vi "Main.vi"() -> ()   [LabVIEW 2018]
doc: "This Continuous Measurement sample project is based on the Queued Message Handler template.\n\nThe Event Handling Loop generates messages based on user interface actions.\n\nThe Message Handling Loop processes messages generated by the Event Handling Loop, or by other messages. There are also Acquisition and Logging message handling loop subVIs, and a chart updating loop."
uses:
  Settings/Settings.ctl
  Acquisition/Hardware Configuration.ctl
  Logging/Logging Configuration.ctl
  controls/UI Data.ctl
  controls/UI State.ctl
  support/Message Queue/Enqueue Message (Single).vi
  support/Message Queue/Enqueue Message (Array).vi
  <vilib>/Utility/error.llb/Error Cluster From Error Code.vi
  <vilib>/ErrorRing/Error Ring.xnode
  Acquisition/Acquisition.lvlib
  Logging/Logging.lvlib
  Settings/Settings.lvlib
  support/User Event - Stop/User Event - Stop.lvlib
  support/Message Queue/Message Queue.lvlib
  Settings/Settings Dialog.vi
panel:
  in  "Data 2":u32(graph)
  out "Config":T1={"Hardware Configuration"={"DAQmx Channel 1"="SimDev1/ai0", "DAQmx Channel 2"="SimDev1/ai1", "DAQmx Channel 3"="SimDev1/ai2", "DAQmx AI Task"="", "Channel 1 Name"="Battery Voltage", "Channel 2 Name"="Battery Current", "Channel 3 Name"="Brake torque", "Sample time"=50, "Samples per second"=1000.0, "Sample mode"=0, "Samples per channel"=0, "Offset Channel 1"=0.0, "Offset Channel 2"=0.0, "Offset Channel 3"=0.0, "Scale Channel 1"=0.0, "Scale Channel 2"=0.0, "Scale Channel 3"=0.0, "DAQmx Counter Channel"="", "Counter Name"="", "DAQmx Counter Task"=""}, "Logging Configuration"={"Log File Base Path"=path "", "TDMS File Reference"=refnum}} {"Hardware Configuration"."Sample mode" items=["Continuous Samples"=10123]}
  out "Data":u32(graph)
  in  "Start":bool
  in  "Stop":bool
  in  "Settings":bool
  out "Status":string
  in  "data to matlab":bool
  in  "Exit":bool
  # "Scooter measurement data"
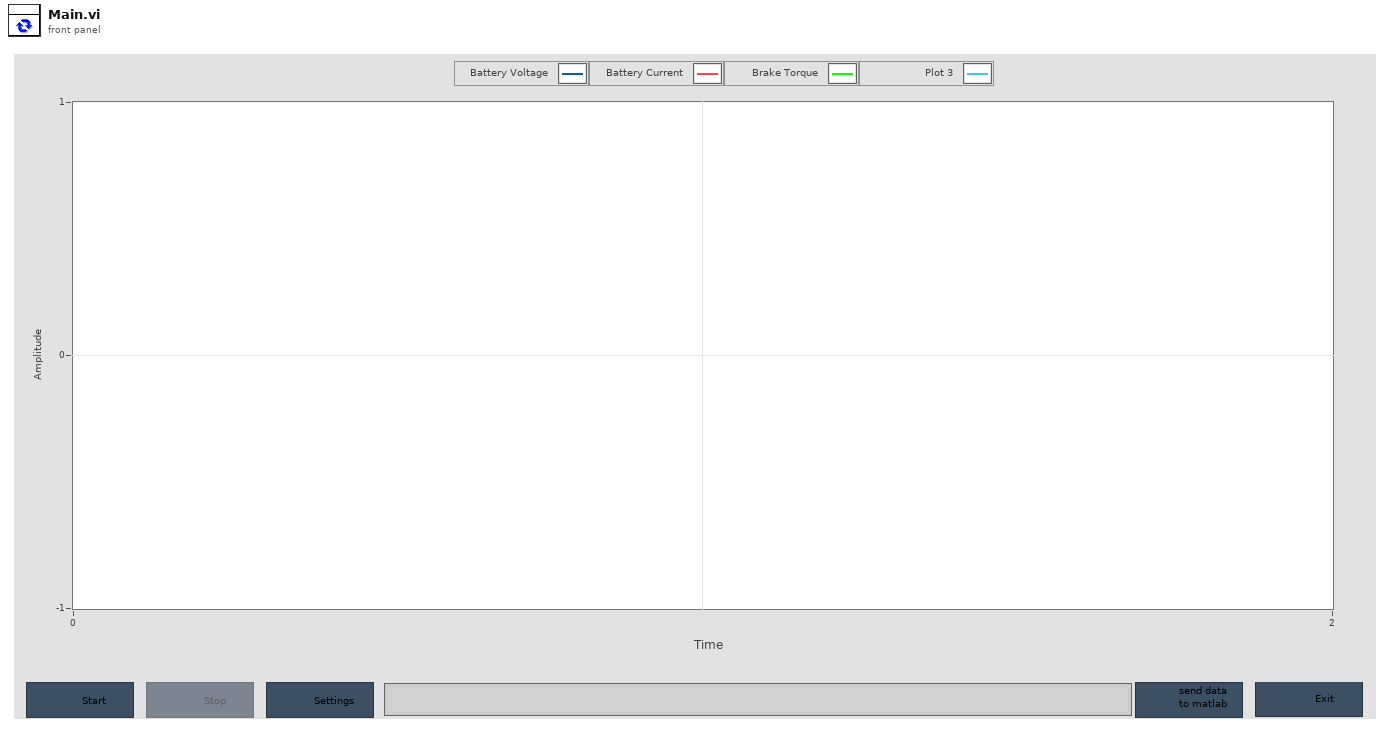
[diagram p1: front panel]
types:
  T1 = typedef "Settings.lvlib/Settings.ctl" = cluster{"Hardware Configuration":T2, "Logging Configuration":T3}
  T2 = typedef "Acquisition.lvlib/Hardware Configuration.ctl" = cluster{"DAQmx Channel 1":tag, "DAQmx Channel 2":tag, "DAQmx Channel 3":tag, "DAQmx AI Task":refnum<k21>, "Channel 1 Name":string, "Channel 2 Name":string, "Channel 3 Name":string, "Sample time":u32, "Samples per second":dbl, "Sample mode":u16, "Samples per channel":i32, "Offset Channel 1":dbl, "Offset Channel 2":dbl, "Offset Channel 3":dbl, "Scale Channel 1":dbl, "Scale Channel 2":dbl, "Scale Channel 3":dbl, "DAQmx Counter Channel":tag, "Counter Name":string, "DAQmx Counter Task":refnum<k21>}
  T3 = typedef "Logging.lvlib/Logging Configuration.ctl" = cluster{"Log File Base Path":path, "TDMS File Reference":refnum<k34>}
  T4 = typedef "UI State.ctl" = enum16{"Idle", "Acquiring and Logging", "Waiting for Exit", "Waiting for Exit (Acq Stopped)", "Waiting for Exit (Log Stopped)", "Waiting for Stop", "Waiting for Stop (Acq Stopped)", "Waiting for Stop (Log Stopped)"}
  T5 = typedef "UI Data.ctl" = cluster{"Start Ref":refnum<vi>, "Stop Ref":refnum<vi>, "Settings Ref":refnum<vi>, "Exit Ref":refnum<vi>, "Status Ref":refnum<vi>, "Data Ref":refnum<vi>, "data to matlab Ref":refnum<vi>}
  T6 = typedef "Message Queue.lvlib/All Message Queues.ctl" = cluster{"UI":refnum<queue>, "Acquisition":refnum<queue>, "Logging":refnum<queue>}
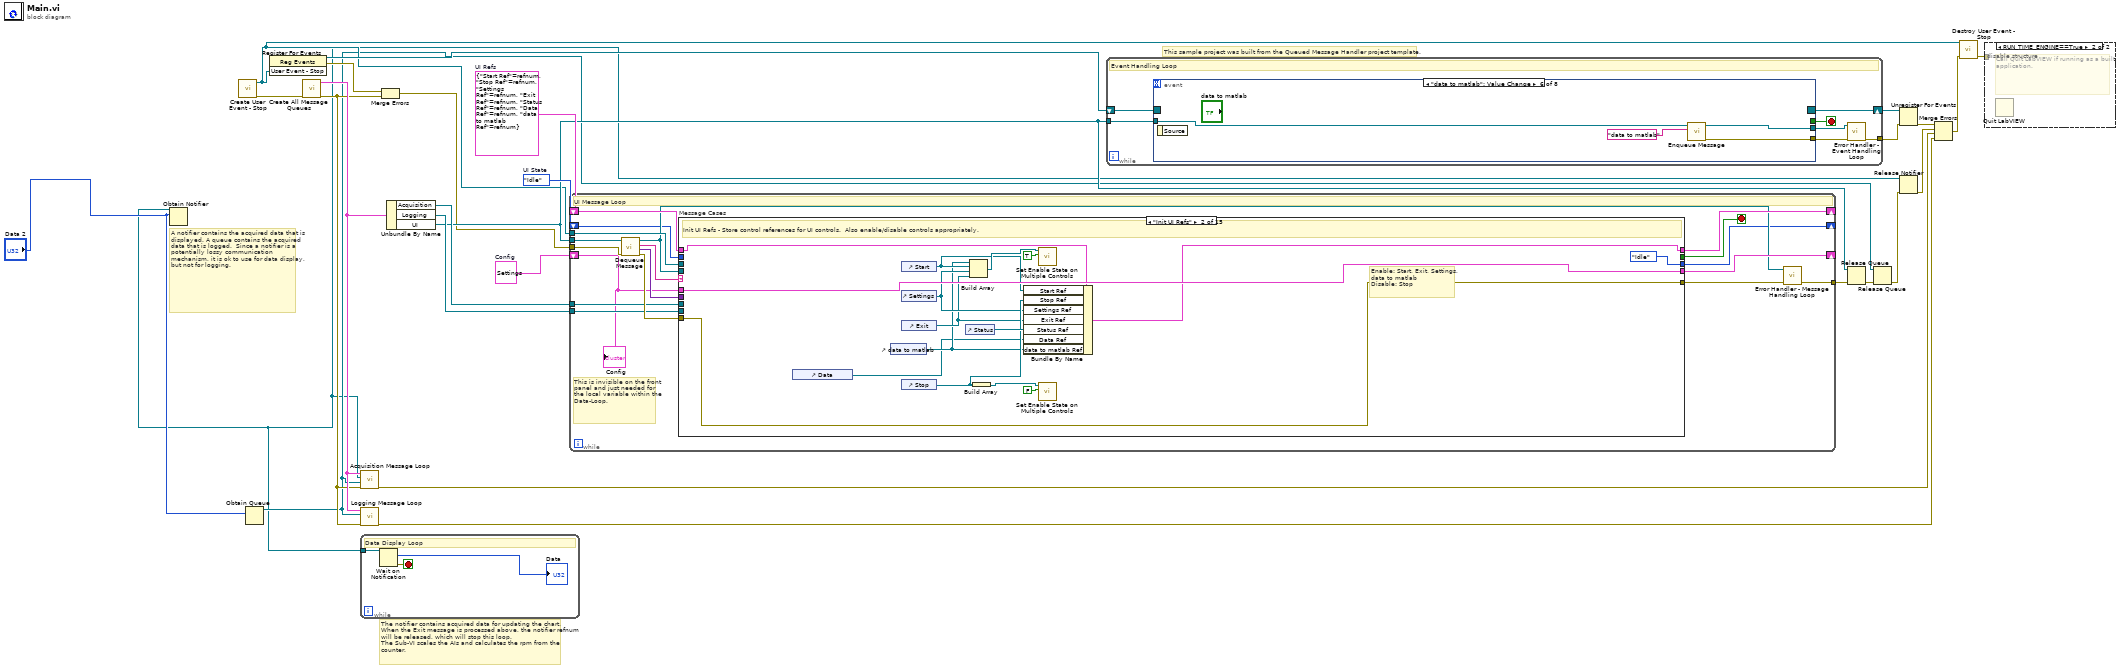
[diagram p0: block diagram]
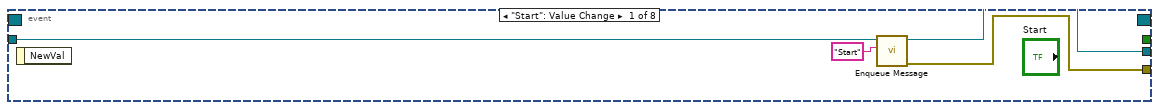
[diagram p3: hidden frame]
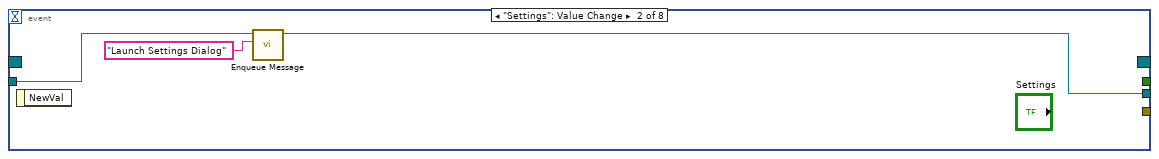
[diagram p4: hidden frame]
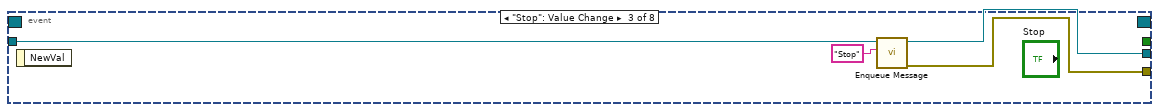
[diagram p5: hidden frame]
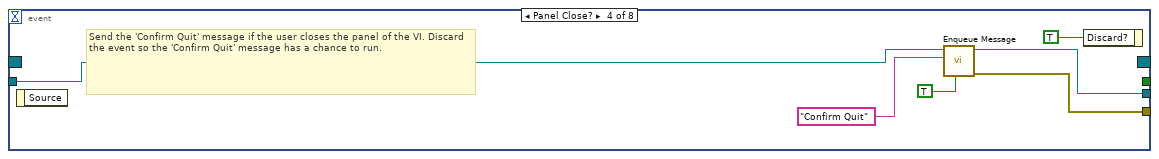
[diagram p6: hidden frame]
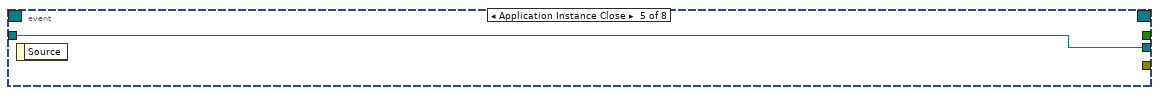
[diagram p7: hidden frame]
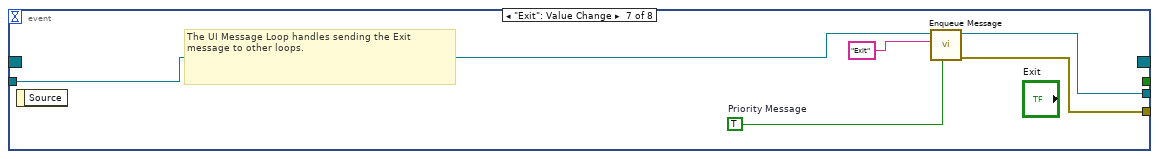
[diagram p8: hidden frame]
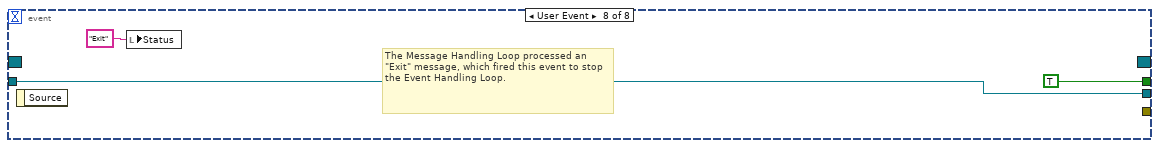
[diagram p9: hidden frame]
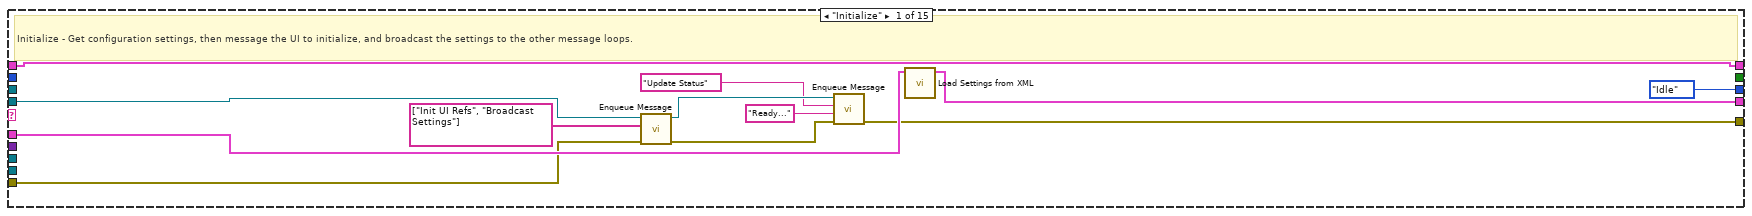
[diagram p10: hidden frame]
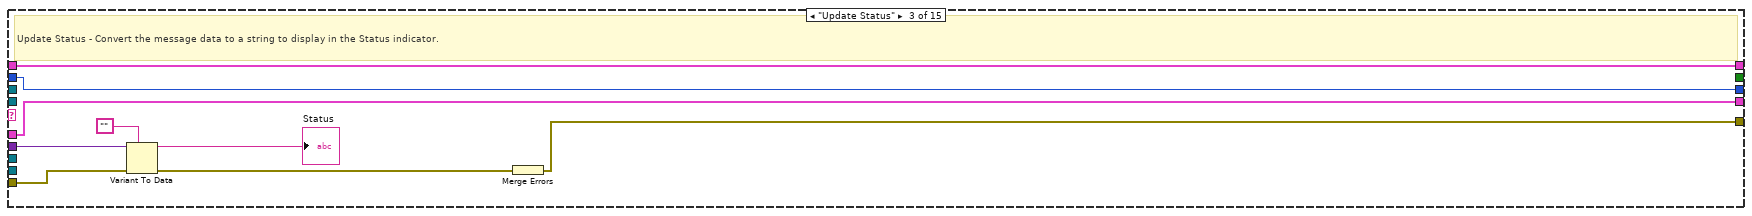
[diagram p11: hidden frame]
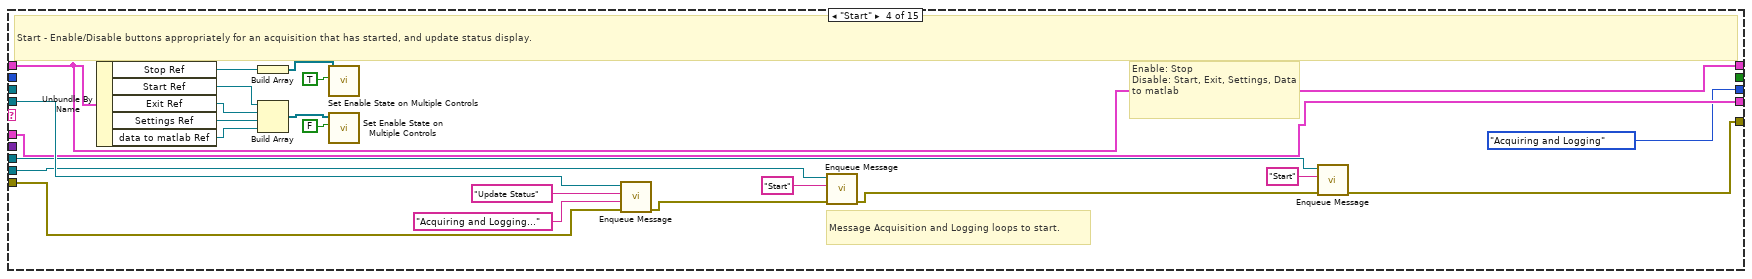
[diagram p12: hidden frame]
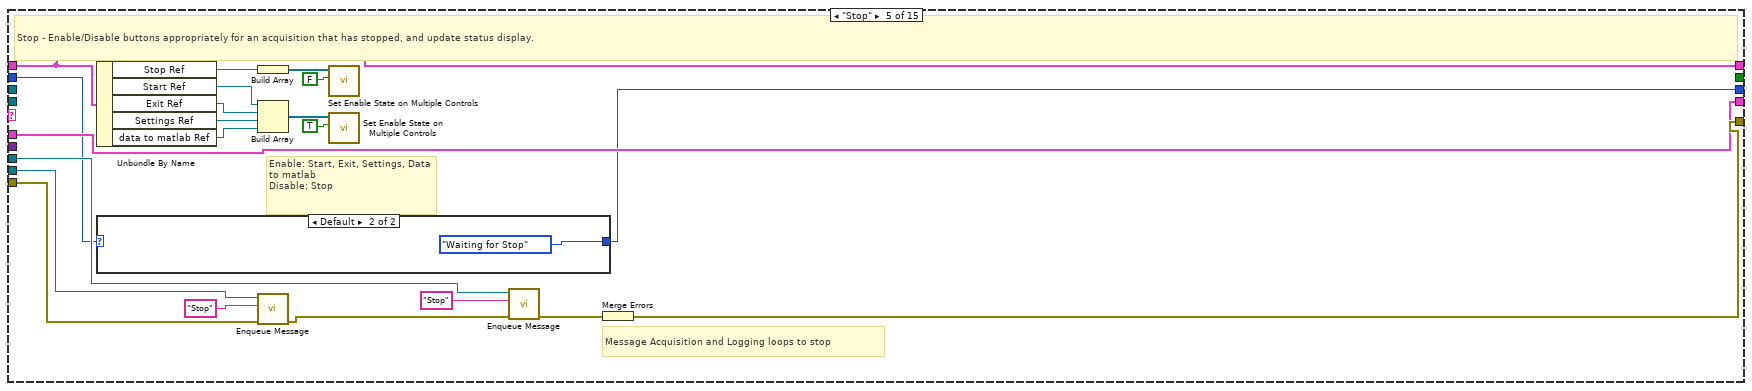
[diagram p13: hidden frame]
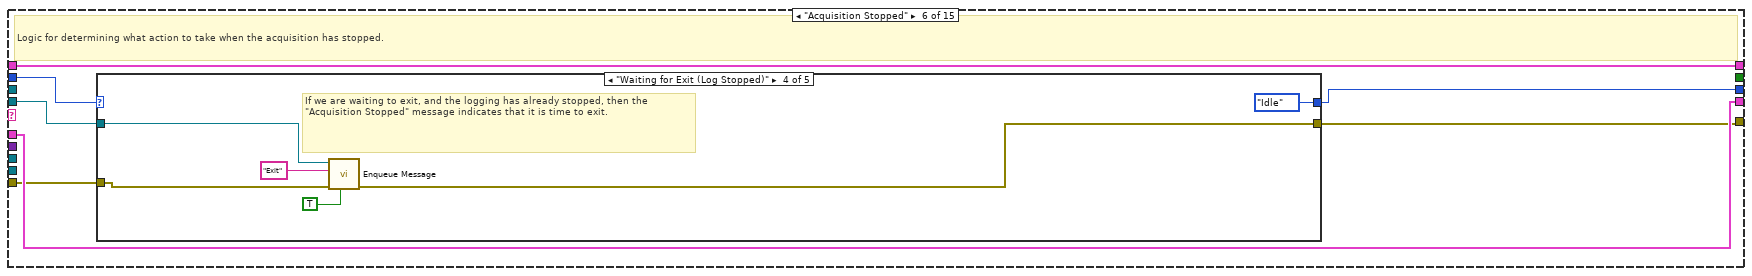
[diagram p15: hidden frame]
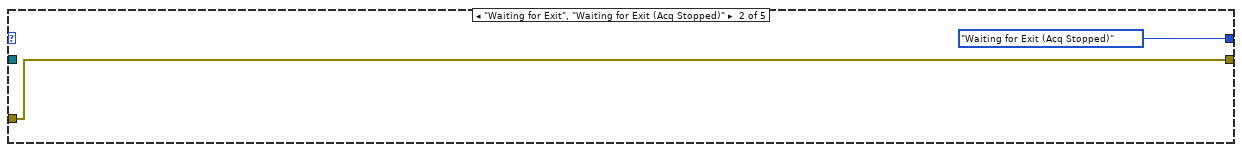
[diagram p17: hidden frame]
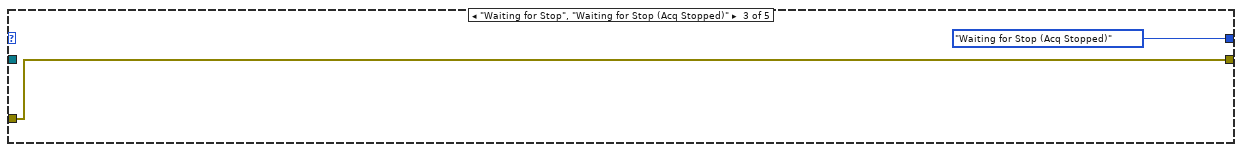
[diagram p18: hidden frame]
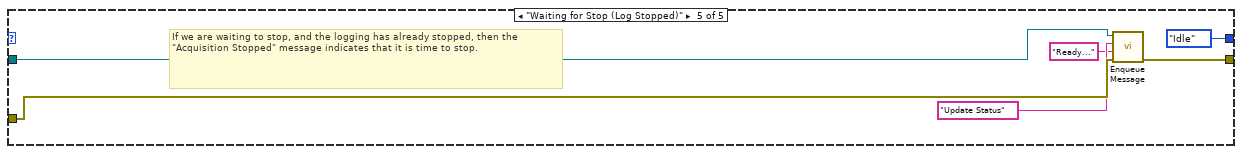
[diagram p19: hidden frame]
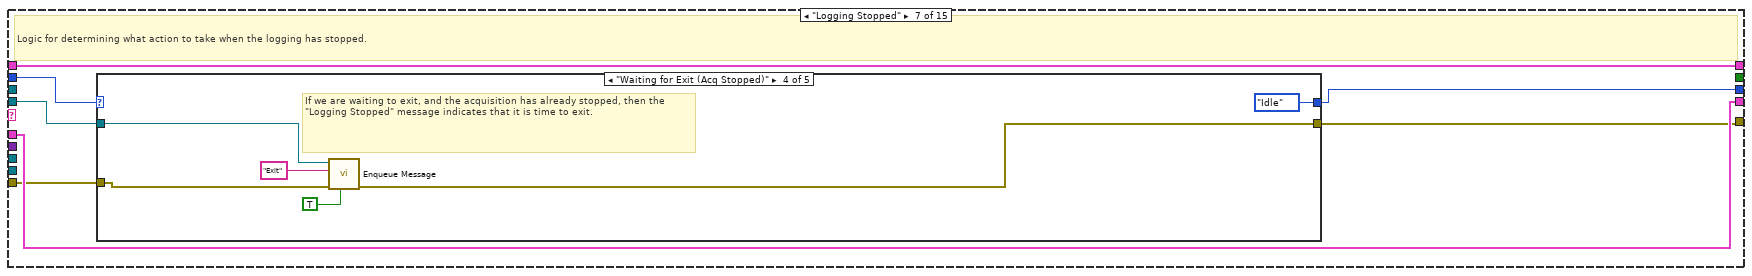
[diagram p20: hidden frame]
diagram:
  w15 = UI_State."Idle"  # UI State
  w18 = T5 {"Start Ref"=refnum, "Stop Ref"=refnum, "Settings Ref"=refnum, "Exit Ref"=refnum, "Status Ref"=refnum, "Data Ref"=refnum, "data to matlab Ref"=refnum}  # UI Refs
  w4 = T1 {"Hardware Configuration"={"DAQmx Channel 1"="", "DAQmx Channel 2"="", "DAQmx Channel 3"="", "DAQmx AI Task"="", "Channel 1 Name"="Battery Voltage", "Channel 2 Name"="Battery Current", "Channel 3 Name"="Brake torque", "Sample time"=50, "Samples per second"=1000.0, "Sample mode"=0, "Samples per channel"=0, "Offset Channel 1"=0.0, "Offset Channel 2"=0.0, "Offset Channel 3"=0.0, "Scale Channel 1"=0.0, "Scale Channel 2"=0.0, "Scale Channel 3"=0.0, "DAQmx Counter Channel"="", "Counter Name"="", "DAQmx Counter Task"=""}, "Logging Configuration"={"Log File Base Path"=path "", "TDMS File Reference"=refnum}}  # Config
  # "This sample project was built from the Queued Message Handler project template."
  # "A notifier contains the acquired data that is displayed. A queue contains the acquired data that is logged.  Since a notifier is a potentially lossy communication mechanism, it is ok to use for data display, but not for logging."
  # "The notifier contains acquired data for updating the chart. When the Exit message is processed above, the notifier refnum will be released, which will stop this loop.\nThe Sub-VI scales the AIs and calculates the rpm from the counter."
  n1 = Obtain Notifier(notification data type="Data 2") -> (notifier out=w1:refnum<notifier>)  [unwired: 3 in, 2 out]
  n2 = call "Create User Event - Stop.vi"() -> ("error out"=w24:errorcluster, "User Event - Stop"=w7:refnum<user-event>)  [unwired: 10 in]
  n3 = Obtain Queue(element data type="Data 2") -> (queue out=w2:refnum<queue>)  [unwired: 4 in, 2 out]
  n4 = register-events(w7) -> (reference out=w8:refnum<event-registration>, error out=w5:errorcluster)  [unwired: 2 in]
  n5 = call "Create All Message Queues.vi"("error in (no error)"=w24) -> ("error out"=w21:errorcluster, "Message Queues out"=w23:T6)  [unwired: 9 in]
  n6 = call "Acquisition Message Loop.vi"("error in (no error)"=w21, "Data Queue"=w2, "Data Notifier"=w1, "Message Queues"=w23) -> ("error out"=w25:errorcluster)  [unwired: 7 in]
  n7 = call "Logging Message Loop.vi"("error in (no error)"=w21, "Data Queue"=w2, "Message Queues"=w23) -> ("error out"=w22:errorcluster)  [unwired: 8 in]
  n8 = while "Data Display Loop" {
    tunnel: w1 -> [w30]
    stop <- w29 stop-if-true
    # "Data Display Loop"
    n9 = Wait on Notification(notifier=w30) -> (notification=→"Data":u32, error out=w29:errorcluster)  [unwired: 3 in, 2 out]
  }
  n10 = Merge Errors(w5, w21) -> (w6:errorcluster)
  n11 = Unbundle By Name(w23) -> ("Acquisition"=w17:refnum<queue>, "Logging"=w16:refnum<queue>, "UI"=w13:refnum<queue>)
  n12 = while {
    tunnel: w13 -> [w42]
    tunnel: w7 -> [w47]
    shift-right: [w41] -> _
    shift-left: w4 -> [w31]
    shift-right: [w39] -> _
    shift-left: w18 -> [w40]
    tunnel: w17 -> [w38]
    tunnel: w16 -> [w37]
    shift-right: [w32] -> _
    shift-left: w15 -> [w33]
    tunnel: w6 -> [w46]
    tunnel: [w36] -> w27
    stop <- w48 stop-if-true
    # "This is invisible on the front panel and just needed for the local variable within the Data-Loop."
    # "UI Message Loop"
    n13 = call "Dequeue Message.vi"("error in (no error)"=w46, "Message Queue"=w42) -> ("error out"=w45:errorcluster, "Message Data"=w43:variant, "Message"=w44:string, "dup Message Queue"=w34:refnum<queue>)  [unwired: 6 in]
    n14 = case "Message Cases" shown="\"Init UI Refs\"" w44 {
      selector: w44 -> [_ _ _ _ _ _ _ _ _ _ _ _ _ _ w273]
      tunnel: w34 -> [w52 _ _ w108 _ w134 w159 _ w199 _ w220 _ _ _ _]
      tunnel: w45 -> [w51 w76 w84 w107 w128 w135 w160 w187 w201 w208 w219 w248 w265 w271 _]
      tunnel: [w56 w76 w85 w90 w129 w132 w157 w193 w194 w211 w218 w258 w264 w266 w272] -> w35
      tunnel: [_ _ _ _ _ _ _ _ _ _ _ TRUE _ _ _] -> w48
      tunnel: w43 -> [_ _ w83 _ _ _ _ _ _ w212 _ w246 _ _ _]
      tunnel: w47 -> [_ _ _ _ _ _ _ _ _ _ _ w259 _ _ _]
      tunnel: [w59 w75 w79 w106 w127 w138 w163 w191 w198 w216 w223 w257 w263 w268 w276] -> w41
      tunnel: w31 -> [w60 w75 w79 w106 w127 w138 w163 w191 w202 w216 w223 w257 w263 w268 w276]
      tunnel: w40 -> [w53 w74 w78 w103 w126 w137 w162 w185 w196 w215 w222 w256 w262 w270 w275]
      tunnel: [w53 w72 w78 w103 w126 w137 w162 w185 w196 w215 w222 w256 w262 w270 w275] -> w39
      tunnel: w38 -> [_ _ _ w89 w113 _ _ w184 _ _ _ w255 _ _ _]
      tunnel: w37 -> [_ _ _ w92 w116 _ _ w183 _ _ _ w254 _ _ _]
      tunnel: w33 -> [_ _ w77 _ w110 w136 w161 w182 w195 w210 w221 _ w261 w269 w274]
      tunnel: [UI_State."Idle" ("UI State") UI_State."Idle" ("UI State") w77 UI_State."Acquiring and Logging" ("UI State") w111 w133 w158 w182 w195 w210 w217 UI_State."Idle" ("UI State") w261 w269 w274] -> w32
      frame "Initialize" {
        # "Initialize - Get configuration settings, then message the UI to initialize, and broadcast the settings to the other message loops."
        n15 = call-poly "Enqueue Message.vi"("error in (no error)"=w51, "Message Array"=string[] ["Init UI Refs", "Broadcast Settings"], "Message Queue"=w52) -> ("error out"=w58:errorcluster, "dup Message Queue"=w57:refnum<queue>)  [unwired: 7 in]
        n16 = call-poly "Enqueue Message.vi"("error in (no error)"=w58, "Message Data"="Ready..." ("Ready..."), "Message"="Update Status", "Message Queue"=w57) -> ("error out"=w56:errorcluster)  [unwired: 6 in, 1 out]
        n17 = call "Load Settings from XML.vi"("Settings in"=w60) -> ("Settings out"=w59:T1)  [unwired: 9 in, 1 out]
      }
      frame "Init UI Refs" {
        # "Enable: Start, Exit, Settings, data to matlab\nDisable: Stop"
        # "Init UI Refs - Store control references for UI controls.  Also enable/disable controls appropriately."
        n18 = control-ref of="Data"() -> (w61:refnum<vi>)
        n19 = control-ref of="data to matlab"() -> (w62:refnum<vi>)
        n20 = control-ref of="Start"() -> (w66:refnum<vi>)
        n21 = control-ref of="Settings"() -> (w65:refnum<vi>)
        n22 = control-ref of="Exit"() -> (w64:refnum<vi>)
        n23 = control-ref of="Stop"() -> (w67:refnum<vi>)
        n24 = control-ref of="Status"() -> (w73:refnum<vi>)
        n25 = Build Array(w62, w66, w65, w64) -> (w70:refnum<vi>[])
        n26 = Build Array(w67) -> (w69:refnum<vi>[])
        n27 = Bundle By Name(cluster=w74, "Start Ref"=w66, "Stop Ref"=w67, "Settings Ref"=w65, "Exit Ref"=w64, "Status Ref"=w73, "Data Ref"=w61, "data to matlab Ref"=w62) -> (w72:T5)
        n28 = call "Set Enable State on Multiple Controls.vi"("Enable?"=TRUE, "Controls"=w70) -> ()  [unwired: 10 in]
        n29 = call "Set Enable State on Multiple Controls.vi"("Enable?"=FALSE, "Controls"=w69) -> ()  [unwired: 10 in]
      }
      frame "Update Status" {
        # "Update Status - Convert the message data to a string to display in the Status indicator."
        n30 = Variant To Data(error in=w84, type="", Variant=w83) -> (data=→"Status":string, error out=w81:errorcluster)
        n31 = Merge Errors(w81) -> (w85:errorcluster)
      }
      frame "Start" {
        # "Message Acquisition and Logging loops to start."
        # "Enable: Stop\nDisable: Start, Exit, Settings, Data to matlab"
        # "Start - Enable/Disable buttons appropriately for an acquisition that has started, and update status display."
        n32 = Unbundle By Name(w103) -> ("Stop Ref"=w98:refnum<vi>, "Start Ref"=w97:refnum<vi>, "Exit Ref"=w96:refnum<vi>, "Settings Ref"=w95:refnum<vi>, "data to matlab Ref"=w86:refnum<vi>)
        n33 = Build Array(w98) -> (w100:refnum<vi>[])
        n34 = Build Array(w97, w96, w95, w86) -> (w101:refnum<vi>[])
        n35 = call "Set Enable State on Multiple Controls.vi"("Enable?"=TRUE, "Controls"=w100) -> ()  [unwired: 10 in]
        n36 = call "Set Enable State on Multiple Controls.vi"("Enable?"=FALSE, "Controls"=w101) -> ()  [unwired: 10 in]
        n37 = call-poly "Enqueue Message.vi"("error in (no error)"=w107, "Message Data"="Acquiring and Logging..." ("Acquiring and Logging..."), "Message"="Update Status", "Message Queue"=w108) -> ("error out"=w94:errorcluster)  [unwired: 6 in, 1 out]
        n38 = call-poly "Enqueue Message.vi"("error in (no error)"=w94, "Message"="Start", "Message Queue"=w92) -> ("error out"=w91:errorcluster)  [unwired: 7 in, 1 out]
        n39 = call-poly "Enqueue Message.vi"("error in (no error)"=w91, "Message"="Start", "Message Queue"=w89) -> ("error out"=w90:errorcluster)  [unwired: 7 in, 1 out]
      }
      frame "Stop" {
        # "Message Acquisition and Logging loops to stop"
        # "Enable: Start, Exit, Settings, Data to matlab\nDisable: Stop"
        # "Stop - Enable/Disable buttons appropriately for an acquisition that has stopped, and update status display."
        n40 = Unbundle By Name(w126) -> ("Stop Ref"=w121:refnum<vi>, "Start Ref"=w120:refnum<vi>, "Exit Ref"=w119:refnum<vi>, "Settings Ref"=w118:refnum<vi>, "data to matlab Ref"=w109:refnum<vi>)
        n41 = case shown="Default" w110 {
          selector: w110 -> [w130 _]
          tunnel: [w130 UI_State."Waiting for Stop" ("UI State")] -> w111
          frame "Waiting for Exit" {
          }
          frame Default {
          }
        }
        n42 = Build Array(w121) -> (w123:refnum<vi>[])
        n43 = Build Array(w120, w119, w118, w109) -> (w124:refnum<vi>[])
        n44 = call-poly "Enqueue Message.vi"("error in (no error)"=w128, "Message"="Stop", "Message Queue"=w116) -> ("error out"=w115:errorcluster)  [unwired: 7 in, 1 out]
        n45 = call "Set Enable State on Multiple Controls.vi"("Enable?"=FALSE, "Controls"=w123) -> ()  [unwired: 10 in]
        n46 = call "Set Enable State on Multiple Controls.vi"("Enable?"=TRUE, "Controls"=w124) -> ()  [unwired: 10 in]
        n47 = call-poly "Enqueue Message.vi"("error in (no error)"=w115, "Message"="Stop", "Message Queue"=w113) -> ("error out"=w114:errorcluster)  [unwired: 7 in, 1 out]
        n48 = Merge Errors(w114) -> (w129:errorcluster)
      }
      frame "Acquisition Stopped" {
        # "Logic for determining what action to take when the acquisition has stopped."
        n49 = case shown="\"Waiting for Exit (Log Stopped)\"" w136 {
          selector: w136 -> [w140 _ _ _ _]
          tunnel: w135 -> [w139 w142 w144 w150 w156]
          tunnel: w134 -> [_ _ _ w148 w153]
          tunnel: [w140 UI_State."Waiting for Exit (Acq Stopped)" ("UI State") UI_State."Waiting for Stop (Acq Stopped)" ("UI State") UI_State."Idle" ("UI State") UI_State."Idle" ("UI State")] -> w133
          tunnel: [w139 w142 w144 w149 w154] -> w132
          frame Default {
          }
          frame "Waiting for Exit", "Waiting for Exit (Acq Stopped)" {
          }
          frame "Waiting for Stop", "Waiting for Stop (Acq Stopped)" {
          }
          frame "Waiting for Exit (Log Stopped)" {
            # "If we are waiting to exit, and the logging has already stopped, then the \"Acquisition Stopped\" message indicates that it is time to exit."
            n50 = call-poly "Enqueue Message.vi"("Priority Message? (F)"=TRUE, "error in (no error)"=w150, "Message"="Exit", "Message Queue"=w148) -> ("error out"=w149:errorcluster)  [unwired: 6 in, 1 out]
          }
          frame "Waiting for Stop (Log Stopped)" {
            # "If we are waiting to stop, and the logging has already stopped, then the \"Acquisition Stopped\" message indicates that it is time to stop."
            n51 = call-poly "Enqueue Message.vi"("error in (no error)"=w156, "Message Data"="Ready..." ("Ready..."), "Message"="Update Status", "Message Queue"=w153) -> ("error out"=w154:errorcluster)  [unwired: 6 in, 1 out]
          }
        }
      }
      frame "Logging Stopped" {
        # "Logic for determining what action to take when the logging has stopped."
        n52 = case shown="\"Waiting for Exit (Acq Stopped)\"" w161 {
          selector: w161 -> [w165 _ _ _ _]
          tunnel: w160 -> [w164 w167 w169 w175 w178]
          tunnel: w159 -> [_ _ _ w173 w177]
          tunnel: [w165 UI_State."Waiting for Exit (Log Stopped)" ("UI State") UI_State."Waiting for Stop (Log Stopped)" ("UI State") UI_State."Idle" ("UI State") UI_State."Idle" ("UI State")] -> w158
          tunnel: [w164 w167 w169 w174 w176] -> w157
          frame Default {
          }
          frame "Waiting for Exit", "Waiting for Exit (Log Stopped)" {
          }
          frame "Waiting for Stop", "Waiting for Stop (Log Stopped)" {
          }
          frame "Waiting for Exit (Acq Stopped)" {
            # "If we are waiting to exit, and the acquisition has already stopped, then the \"Logging Stopped\" message indicates that it is time to exit."
            n53 = call-poly "Enqueue Message.vi"("Priority Message? (F)"=TRUE, "error in (no error)"=w175, "Message"="Exit", "Message Queue"=w173) -> ("error out"=w174:errorcluster)  [unwired: 6 in, 1 out]
          }
          frame "Waiting for Stop (Acq Stopped)" {
            # "If we are waiting to stop, and the acquisition has already stopped, then the \"Logging Stopped\" message indicates that it is time to stop."
            n54 = call-poly "Enqueue Message.vi"("error in (no error)"=w178, "Message Data"="Ready..." ("Ready..."), "Message"="Update Status", "Message Queue"=w177) -> ("error out"=w176:errorcluster)  [unwired: 6 in, 1 out]
          }
        }
      }
      frame "Broadcast settings" {
        w186 = "Update Settings" ("Message")
        # "Broadcast settings - Send the 'Update Settings' message to the Logging and Acquisition message loops."
        n55 = Unbundle By Name(w191) -> ("Hardware Configuration"=w190:T2, "Logging Configuration"=w189:T3)
        n56 = call-poly "Enqueue Message.vi"("Message Data"=w190, "Message"=w186, "Message Queue"=w184) -> ("error out"=w192:errorcluster)  [unwired: 7 in, 1 out]
        n57 = call-poly "Enqueue Message.vi"("error in (no error)"=w192, "Message Data"=w189, "Message"=w186, "Message Queue"=w183) -> ("error out"=w188:errorcluster)  [unwired: 6 in, 1 out]
        n58 = Merge Errors(w188, w187) -> (w193:errorcluster)
      }
      frame "Launch Settings Dialog" {
        # "Launch Settings Dialog - Launch the Settings Dialog when the user clicks the 'Settings' button."
        n59 = call-by-ref "?"("error in (no error)"=w201, "Settings in"=w202) -> ("error out"=w197:errorcluster, "Cancelled?"=w200:bool, "Settings out"=w198:T1)  [unwired: 8 in, 3 out]
        n60 = case shown="False" w200 {
          tunnel: w199 -> [w206 _]
          tunnel: w197 -> [w205 w207]
          tunnel: [w204 w207] -> w194
          frame False {
            n61 = call-poly "Enqueue Message.vi"("error in (no error)"=w205, "Message"="Broadcast Settings", "Message Queue"=w206) -> ("error out"=w204:errorcluster)  [unwired: 7 in, 1 out]
          }
          frame True {
          }
        }
      }
      frame "Error" {
        # "Error - Display an error dialog. This message is sent by the \"Error Handler\" VIs at the end of other loops in this application."
        n62 = Variant To Data(error in=w208, type=errorcluster {"status"=FALSE, "code"=0, "source"=""} ("error constant"), Variant=w212) -> (data=w209:errorcluster, error out=w213:errorcluster)
        n63 = call <vilib>:"Simple Error Handler.vi"("error in (no error)"=w209) -> ()  [unwired: 4 in, 5 out]
        n64 = Merge Errors(w213) -> (w211:errorcluster)
      }
      frame "Confirm Quit" {
        # "Confirm Quit - Message that can confirm whether or not the user wants to exit the application."
        n65 = case shown="\"Acquiring and Logging\"" w221 {
          tunnel: w220 -> [w229 w233]
          tunnel: w219 -> [w228 w232]
          tunnel: [w227 w231] -> w218
          tunnel: [UI_State."Idle" ("UI State") w230] -> w217
          frame Default {
            # "If 'Confirm Quit' comes in while the system is idle, there is no need for a confirmation message."
            n66 = call-poly "Enqueue Message.vi"("Priority Message? (F)"=TRUE, "error in (no error)"=w228, "Message"="Exit", "Message Queue"=w229) -> ("error out"=w227:errorcluster)  [unwired: 6 in, 1 out]
          }
          frame "Acquiring and Logging" {
            n67 = Two Button Dialog(message="Are you sure you want to quit while the acquisition is running?" ("Confirm Quit Message"), 1:"No" ("No"), 2:"Yes" ("Yes")) -> (T button?=w234:bool)
            n68 = case shown="True" w234 {
              tunnel: w233 -> [_ w243]
              tunnel: w232 -> [w239 w244]
              tunnel: [w239 w242] -> w231
              tunnel: [UI_State."Acquiring and Logging" ("UI State") UI_State."Waiting for Exit" ("UI State")] -> w230
              frame False {
                # "User did not want to quit."
              }
              frame True {
                n69 = call-poly "Enqueue Message.vi"("error in (no error)"=w244, "Message"="Stop", "Message Queue"=w243) -> ("error out"=w242:errorcluster)  [unwired: 7 in, 1 out]
              }
            }
          }
        }
      }
      frame "Exit" {
        w250 = TRUE ("Priority Message? (F)")
        w251 = "Exit" ("Message")
        # "Popup an error dialog if 'Exit' was called as a result of an error."
        # "Stop the VI"
        # "Exit - Send Exit messages to the Acquisition and Logging loops, and fire the user event to stop the Event Handling Loop."
        n70 = Variant To Data(type=errorcluster {"status"=FALSE, "code"=0, "source"=""} ("error constant"), Variant=w246) -> (data=w245:errorcluster)  [unwired: 1 in, 1 out]
        n71 = call-poly "Enqueue Message.vi"("Priority Message? (F)"=w250, "error in (no error)"=w248, "Message"=w251, "Message Queue"=w255) -> ("error out"=w252:errorcluster)  [unwired: 6 in, 1 out]
        n72 = call <vilib>:"Simple Error Handler.vi"("error in (no error)"=w245) -> ()  [unwired: 4 in, 5 out]
        n73 = call-poly "Enqueue Message.vi"("Priority Message? (F)"=w250, "error in (no error)"=w252, "Message"=w251, "Message Queue"=w254) -> ("error out"=w249:errorcluster)  [unwired: 6 in, 1 out]
        n74 = call "Fire User Event - Stop.vi"("error in (no error)"=w249, "User Event - Stop"=w259) -> ("error out"=w258:errorcluster)  [unwired: 9 in]
      }
      frame "---Copy This Frame---" {
        # "Duplicate this frame when creating new messages.  Change this comment in the duplicated frame to describe this message."
        n75 = Merge Errors(w265) -> (w264:errorcluster)
      }
      frame "data to matlab" {
        # "reads the tdms-file from settings, splits the signal into inputs and time, converts the timearray to relative time and forwards the variables to matlab for further inspection"
        n76 = Merge Errors(w271) -> (w267:errorcluster)
        n77 = call "data-to-matlab.vi"("error in (no error)"=w267, "Config"=w268) -> ("error out"=w266:errorcluster)  [unwired: 9 in]
      }
      frame Default {
        # "'Default' case only runs if there is a message that isn't defined in any of the other cases.  Output a programming error."
        n78 = xnode "Error Ring"("parameter 0"=w273) -> ("error out"=w272:errorcluster)
      }
    }
    n79 = call "Error Handler - Message Handling Loop.vi"("error in (no error)"=w35, "Message Queue"=w34) -> ("dup error in"=w36:errorcluster)  [unwired: 8 in, 1 out]
    "Config" <- w31
  }
  n80 = while {
    tunnel: w13 -> [w289]
    tunnel: [w286] -> w26
    shift-right: [w288] -> w19
    shift-left: w8 -> [w290]
    stop <- w287 stop-if-true
    # "Event Handling Loop"
    n81 = event shown="[5] \"data to matlab\": Value Change" {
      selector: w290 -> [_ _ _ _ _ _ _ _]
      dyn-events: [_ _ _ _ _ _ _ _] -> w288
      timeout: _ -> [_ _ _ _ _ _ _ _]
      tunnel: [_ _ _ _ _ _ _ TRUE ("Discard?")] -> w287
      tunnel: w289 -> [w294 w296 w300 w305 w308 w312 w314 w318]
      tunnel: [w292 _ w299 w303 _ w310 w317 _] -> w285
      tunnel: [w291 w295 w298 w304 w308 w311 w313 w318] -> w284
      event "Start": Value Change {
        n82 = event-data() -> ()  [unwired: 1 in, 1 out]
        n83 = call-poly "Enqueue Message.vi"("Message"="Start", "Message Queue"=w294) -> ("error out"=w292:errorcluster, "dup Message Queue"=w291:refnum<queue>)  [unwired: 8 in]
      }
      event "Settings": Value Change {
        n84 = event-data() -> ()  [unwired: 1 in, 1 out]
        n85 = call-poly "Enqueue Message.vi"("Message"="Launch Settings Dialog", "Message Queue"=w296) -> ("dup Message Queue"=w295:refnum<queue>)  [unwired: 8 in, 1 out]
      }
      event "Stop": Value Change {
        n86 = event-data() -> ()  [unwired: 1 in, 1 out]
        n87 = call-poly "Enqueue Message.vi"("Message"="Stop", "Message Queue"=w300) -> ("error out"=w299:errorcluster, "dup Message Queue"=w298:refnum<queue>)  [unwired: 8 in]
      }
      event Panel Close? {
        # "Send the 'Confirm Quit' message if the user closes the panel of the VI. Discard the event so the 'Confirm Quit' message has a chance to run."
        n88 = event-data() -> ()  [unwired: 1 in, 1 out]
        n89 = call-poly "Enqueue Message.vi"("Priority Message? (F)"=TRUE, "Message"="Confirm Quit", "Message Queue"=w305) -> ("error out"=w303:errorcluster, "dup Message Queue"=w304:refnum<queue>)  [unwired: 7 in]
        n90 = event-data("Discard?"=TRUE) -> ()  [unwired: 1 in, 1 out]
      }
      event Application Instance Close {
        n91 = event-data() -> ()  [unwired: 1 in, 1 out]
      }
      event "data to matlab": Value Change {
        n92 = event-data() -> ()  [unwired: 1 in, 1 out]
        n93 = call-poly "Enqueue Message.vi"("Message"="data to matlab", "Message Queue"=w312) -> ("error out"=w310:errorcluster, "dup Message Queue"=w311:refnum<queue>)  [unwired: 8 in]
      }
      event "Exit": Value Change {
        w315 = TRUE  # Priority Message
        # "The UI Message Loop handles sending the Exit message to other loops."
        n94 = event-data() -> ()  [unwired: 1 in, 1 out]
        n95 = call-poly "Enqueue Message.vi"("Priority Message? (F)"=w315, "Message"="Exit", "Message Queue"=w314) -> ("error out"=w317:errorcluster, "dup Message Queue"=w313:refnum<queue>)  [unwired: 7 in]
      }
      event User Event {
        # "The Message Handling Loop processed an \"Exit\" message, which fired this event to stop the Event Handling Loop."
        n96 = event-data() -> ()  [unwired: 1 in, 1 out]
        n97 = local write "Status"("Exit" ("Exit String")) -> ()
      }
    }
    n98 = call "Error Handler - Event Handling Loop.vi"("error in (no error)"=w285, "Message Queue"=w284) -> ("dup error in"=w286:errorcluster)  [unwired: 8 in, 1 out]
  }
  n99 = Release Queue(queue=w13, error in (no error)=w27) -> (error out=w11:errorcluster)  [unwired: 1 in, 2 out]
  n100 = Release Queue(queue=w2, error in (no error)=w11) -> (error out=w10:errorcluster)  [unwired: 1 in, 2 out]
  n101 = Unregister For Events(event registration refnum=w19, error in=w26) -> (error out=w20:errorcluster)
  n102 = Release Notifier(notifier=w1, error in (no error)=w10) -> (error out=w9:errorcluster)  [unwired: 1 in, 2 out]
  n103 = Merge Errors(w20, w9, w25, w22) -> (w14:errorcluster)
  n104 = call "Destroy User Event - Stop.vi"("error in (no error)"=w14, "User Event - Stop"=w7) -> ("error out"=w12:errorcluster)  [unwired: 9 in]
  n105 = disable-structure shown="RUN_TIME_ENGINE==True" {
    disable-tunnel: w12 -> [_ _]
    frame condition #0 (active) {
    }
    frame condition #1 {
      # "Call Quit LabVIEW if running as a built application."
      n106 = Quit LabVIEW() -> ()  [unwired: 1 in]
    }
  }
